vi "DigitalOut_2.vi"(8 "Purge Valves":bool[](array[boolean])=[FALSE, FALSE], 10 "Spark Arm":bool, 11 "Ignition!":bool) -> (0 "purge valves out":bool[](array[boolean]))   [LabVIEW 2018]
uses:
  3a15f5c1-9116-443e-bdb1-33a1cd757f7d.vi
  <vilib>/DAQmx/write.llb/DAQmx Write (Digital 1D Bool NChan 1Samp 1Line).vi
  <vilib>/DAQmx/create/channels.llb/DAQmx Create Channel (CO-Pulse Generation-Frequency).vi
  <vilib>/DAQmx/configure/timing.llb/DAQmx Timing (Implicit).vi
  <vilib>/DAQmx/miscellaneous.llb/DAQmx Fill In Error Info.vi
  <resource>/objmgr/daqmx.rc
panel:
  # "NC-FP"
  # "NC-OP"
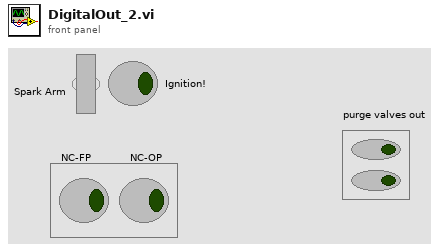
[diagram p1: front panel]
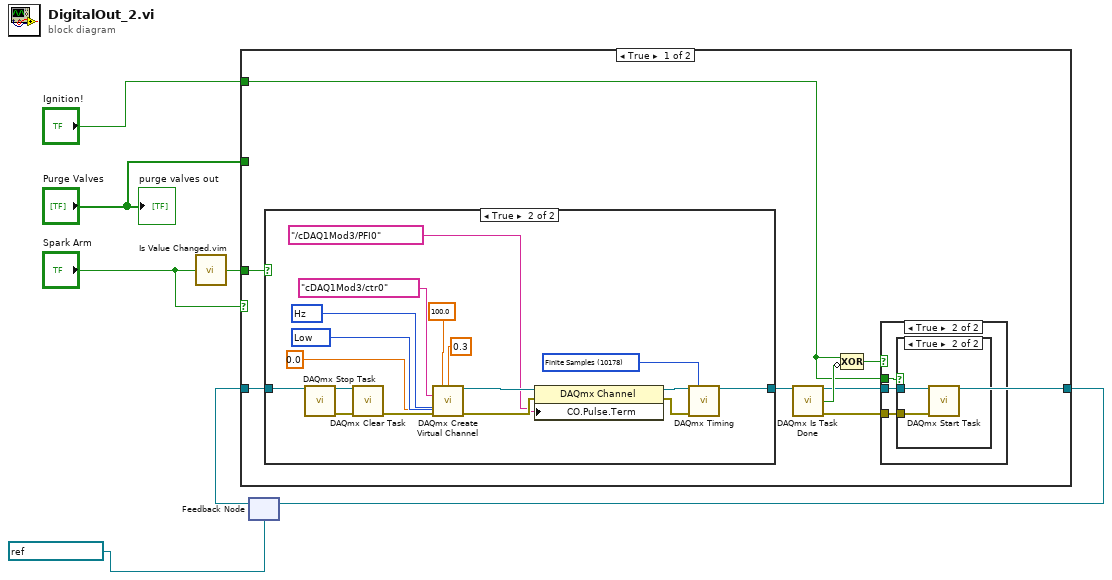
[diagram p0: block diagram]
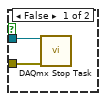
[diagram p3: hidden frame]
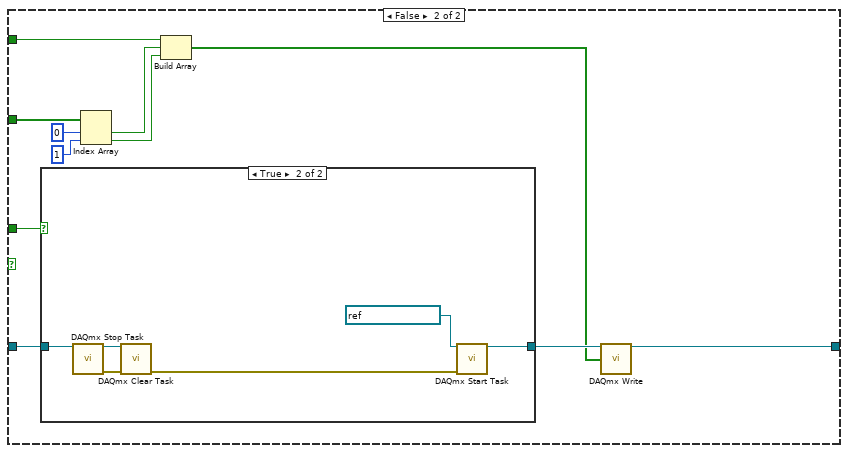
[diagram p5: hidden frame]
diagram:
  n1 = call "Is Value Changed.vim"("value"="Spark Arm") -> ("changed or first call?"=w6:bool)
  n2 = feedback #1(refnum<k21> "Dout2 Task" ("task in")) -> (w3:refnum<k21>)
  n3 = case shown="True" "Spark Arm" {
    tunnel: w6 -> [w8 w42]
    tunnel: "Purge Valves" -> [_ w46]
    tunnel: "Ignition!" -> [w11 w45]
    tunnel: w3 -> [w15 w51]
    tunnel: [w9 w49] -> w2
    frame True {
      n4 = case shown="True" w8 {
        tunnel: w15 -> [w23 w33]
        tunnel: [w23 w32] -> w14
        frame False {
        }
        frame True {
          w34 = 10178 items=["Finite Samples"=10178, "Continuous Samples"=10123, "Hardware Timed Single Point"=12522] ("sample mode")
          w36 = 10214 items=["High"=10192, "Low"=10214] ("idle state")
          w37 = 10373 items=["Hz"=10373] ("units")
          n5 = call <vilib>:"DAQmx Stop Task.vi"("task/channels in"=w33) -> ("task out"=w38:refnum<k21>, "error out"=w39:errorcluster)  [unwired: 13 in]
          n6 = call <vilib>:"DAQmx Clear Task.vi"("task in"=w38, "error in"=w39) -> ("error out"=w40:errorcluster)  [unwired: 13 in]
          n7 = call-poly <vilib>:"DAQmx Create Virtual Channel.vi"("frequency"=100.0, "duty cycle"=0.3, "counter"=tag "cDAQ1Mod3/ctr0", "units"=w37, "error in"=w40, "idle state"=w36, "initial delay"=0.0) -> ("task out"=w31:refnum<k21>, "error out"=w26:errorcluster)  [unwired: 7 in]
          n8 = property class="DAQmx Channel"(reference=w31, error in=w26, "CO.Pulse.Term"=tag "/cDAQ1Mod3/PFI0" ("AIConvClk.OutputTerm")) -> (reference out=w27:refnum<k21>, error out=w25:errorcluster)
          n9 = call-poly <vilib>:"DAQmx Timing.vi"("task/channels in"=w27, "sample mode"=w34, "error in"=w25) -> ("task out"=w32:refnum<k21>)  [unwired: 11 in, 1 out]
        }
      }
      n10 = call <vilib>:"DAQmx Is Task Done.vi"("task/channels in"=w14) -> ("task out"=w9:refnum<k21>, "task done?"=w13:bool, "error out"=w10:errorcluster)  [unwired: 12 in]
      n11 = Compound Arithmetic op=XOR(w11, invert w13) -> (w12:bool)
      n12 = case shown="True" w12 {
        tunnel: w11 -> [_ w18]
        tunnel: w9 -> [_ w17]
        tunnel: w10 -> [_ w16]
        frame False {
        }
        frame True {
          n13 = case shown="True" w18 {
            tunnel: w17 -> [w20 w22]
            tunnel: w16 -> [w19 w21]
            frame False {
              n14 = call <vilib>:"DAQmx Stop Task.vi"("task/channels in"=w20, "error in"=w19) -> ()  [unwired: 12 in, 2 out]
            }
            frame True {
              n15 = call <vilib>:"DAQmx Start Task.vi"("task/channels in"=w22, "error in"=w21) -> ()  [unwired: 12 in, 2 out]
            }
          }
        }
      }
    }
    frame False {
      n16 = case shown="True" w42 {
        tunnel: w51 -> [w52 w56]
        tunnel: [w52 w55] -> w50
        frame False {
        }
        frame True {
          n17 = call <vilib>:"DAQmx Stop Task.vi"("task/channels in"=w56) -> ("task out"=w57:refnum<k21>, "error out"=w58:errorcluster)  [unwired: 13 in]
          n18 = call <vilib>:"DAQmx Clear Task.vi"("task in"=w57, "error in"=w58) -> ("error out"=w53:errorcluster)  [unwired: 13 in]
          n19 = call <vilib>:"DAQmx Start Task.vi"("task/channels in"=refnum<k21> "Dout2 Task" ("task in"), "error in"=w53) -> ("task out"=w55:refnum<k21>)  [unwired: 12 in, 1 out]
        }
      }
      n20 = Index Array(array=w46, index #1=0 ("index"), index #2=1 ("index")) -> (element #1=w44:bool, element #2=w41:bool)
      n21 = Build Array(w45, w44, w41) -> (w43:bool[])
      n22 = call-poly <vilib>:"DAQmx Write.vi"("task/channels in"=w50, "data"=w43) -> ("task out"=w49:refnum<k21>)  [unwired: 11 in, 2 out]
    }
  }
  n23 = feedback-in #1(w2) -> ()
  "purge valves out" <- "Purge Valves"
